vi "Operations.vi"(6 "Current Index":i32, 8 "Error in":errorcluster, 9 "Inport Values":dbl[](array[numeric]), 10 "Outport Values":dbl[](array[numeric]), 11 "Outport Index":i32) -> (0 "error out":errorcluster, 2 "Outport Values":dbl[](array[numeric]))   [LabVIEW 2025, in "Inline HW Engine.lvlib"]
uses:
  Inline HW Engine.lvlib
  HW Operations.ctl
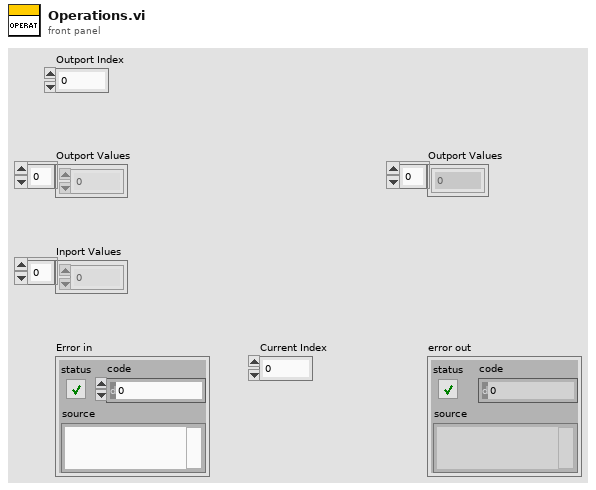
[diagram p1: front panel]
types:
  T1 = typedef "HW Operations.ctl" = enum16{"Initialize", "Set In Val", "Get In Val", "Set Out Val", "Get Out Val", "Get Array"}
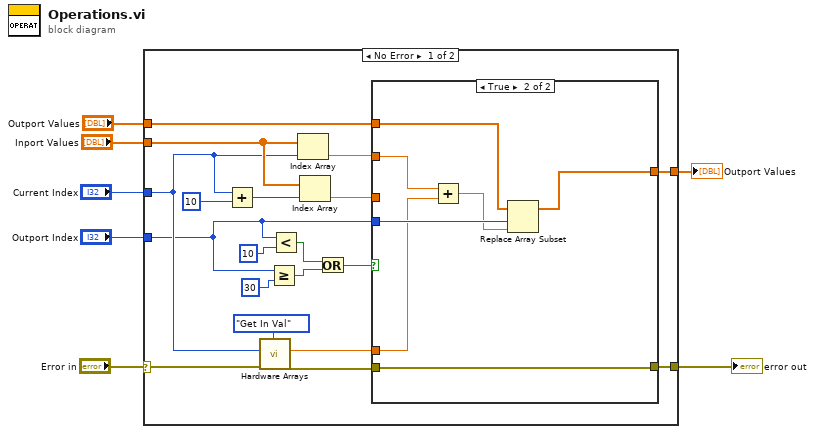
[diagram p0: block diagram]
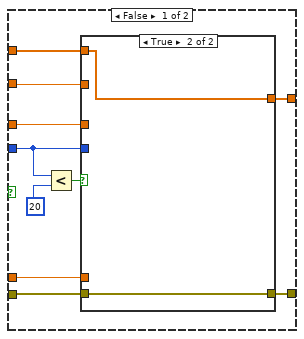
[diagram p2: hidden frame]
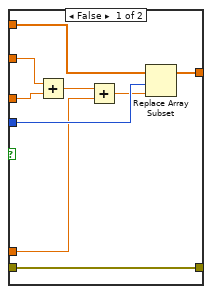
[diagram p3: hidden frame]
diagram:
  n1 = case shown="No Error" "Error in" {
    selector: "Error in" -> [w26 w56]
    tunnel: "Outport Values" -> [w18 w55]
    tunnel: "Inport Values" -> [w14 _]
    tunnel: "Current Index" -> [w9 _]
    tunnel: [w12 w55] -> w2
    tunnel: "Outport Index" -> [w8 _]
    tunnel: [w24 w56] -> w6
    frame No Error {
      n2 = Add(x=w9, y=10) -> (x+y=w15:i32)
      n3 = call "Hardware Arrays.vi"("error in"=w26, "Index"=w9, "Curr Operation"=HW_Operations."Get In Val") -> ("error out"=w25:errorcluster, "Value"=w10:dbl)  [unwired: 5 in, 2 out]
      n4 = Greater Or Equal?(x=w8, y=30) -> (x >= y?=w21:bool)
      n5 = Less?(x=w8, y=10) -> (x < y?=w22:bool)
      n6 = Index Array(array=w14, index=w9) -> (element=w17:dbl)
      n7 = Index Array(array=w14, index=w15) -> (element=w13:dbl)
      n8 = Or(x=w22, y=w21) -> (x .or. y?=w19:bool)
      n9 = case shown="True" w19 {
        tunnel: w18 -> [w31 w53]
        tunnel: w17 -> [w32 w50]
        tunnel: w8 -> [w30 w51]
        tunnel: [w29 w52] -> w12
        tunnel: w13 -> [w28 _]
        tunnel: w25 -> [w36 w54]
        tunnel: [w35 w54] -> w24
        tunnel: w10 -> [w27 w49]
        frame False {
          n10 = Less?(x=w30, y=20) -> (x < y?=w33:bool)
          n11 = case shown="True" w33 {
            tunnel: w32 -> [w42 _]
            tunnel: w31 -> [w44 w46]
            tunnel: w30 -> [w40 _]
            tunnel: [w43 w46] -> w29
            tunnel: w28 -> [w41 _]
            tunnel: w36 -> [w45 w47]
            tunnel: [w45 w47] -> w35
            tunnel: w27 -> [w37 _]
            frame False {
              n12 = Add(x=w42, y=w41) -> (x+y=w38:dbl)
              n13 = Add(x=w38, y=w37) -> (x+y=w39:dbl)
              n14 = Replace Array Subset(array=w44, new element=w39, index=w40) -> (w43:dbl[])
            }
            frame True {
            }
          }
        }
        frame True {
          n15 = Add(x=w50, y=w49) -> (x+y=w48:dbl)
          n16 = Replace Array Subset(array=w53, new element=w48, index=w51) -> (w52:dbl[])
        }
      }
    }
    frame Error {
    }
  }
  "Outport Values" <- w2
  "error out" <- w6
